vi "Execute.vi"(8 "error in":errorcluster, 9 "Path":path, 10 "Name":string) -> (0 "error out":errorcluster)   [LabVIEW 2019, in "Launcher.lvlib" / "Launcher.lvclass"]
uses:
  Library/Launcher.lvclass
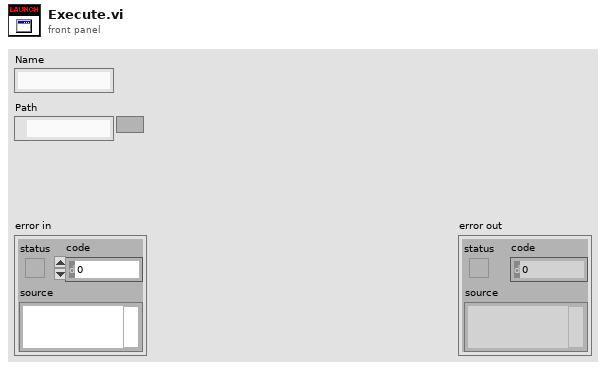
[diagram p1: front panel]
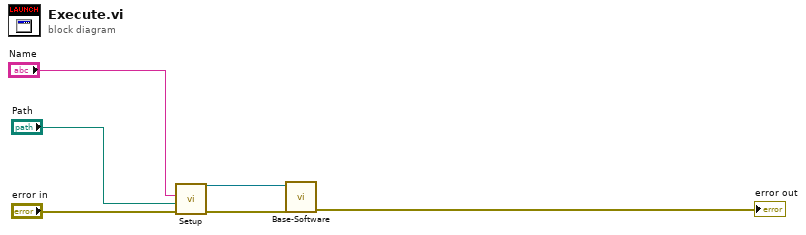
[diagram p0: block diagram]
diagram:
  n1 = call "Setup.vi"("error in"="error in", "Path"="Path", "Name"="Name") -> ("error out"=w4:errorcluster, "Launcher out"=w5:refnum<class "Launcher.lvclass">)  [unwired: 7 in]
  n2 = call "Base-Software.vi"("error in"=w4, "Launcher in"=w5) -> ("error out"=→"error out":errorcluster)  [unwired: 8 in, 1 out]
